vi "clearCategoryDefaultAmount.vi"(8 "error in (no error)":errorcluster, 10 "Name":string, 11 "Account History in":refnum<class "Account History.lvclass">) -> (0 "error out":errorcluster, 3 "Account History out":refnum<class "Account History.lvclass">)   [LabVIEW 2018, in "Account History.lvclass"]
uses:
  Account History.lvclass
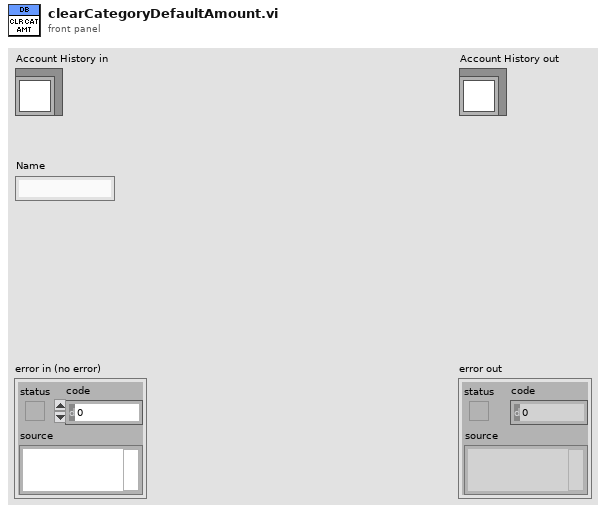
[diagram p1: front panel]
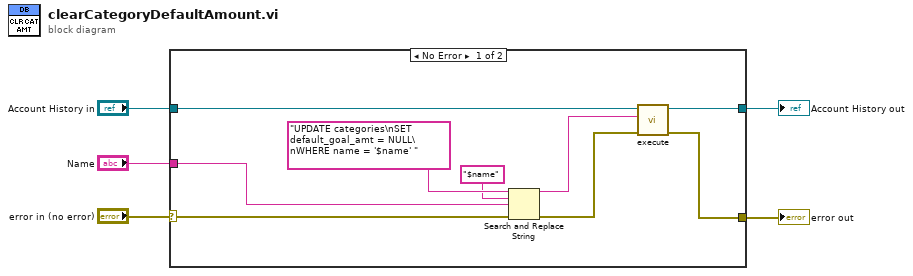
[diagram p0: block diagram]
diagram:
  n1 = case shown="No Error" "error in (no error)" {
    selector: "error in (no error)" -> [w7 w16]
    tunnel: [w10 w16] -> w4
    tunnel: [w11 w15] -> w2
    tunnel: "Account History in" -> [w12 w15]
    tunnel: "Name" -> [w6 _]
    frame No Error {
      n2 = Search and Replace String(input string="UPDATE categories\nSET default_goal_amt = NULL\nWHERE name = '$name' ", search string="$name", replace string=w6, error in=w7) -> (result string=w9:string, error out=w8:errorcluster)  [unwired: 4 in, 2 out]
      n3 = call "execute.vi"("error in (no error)"=w8, "SQL query"=w9, "Database in"=w12) -> ("error out"=w10:errorcluster, "Database out"=w11:refnum<class "Account History.lvclass">)  [unwired: 7 in]
    }
    frame Error {
    }
  }
  "error out" <- w4
  "Account History out" <- w2
